vi "Wait For Motion.vi"(8 "error in":errorcluster, 10 "Axes":string[](array[string])=["X", "Y", "Z", "U"], 11 "Gantry in":refnum<class "Gantry.lvclass">) -> (0 "error out":errorcluster, 3 "Gantry out":refnum<class "Gantry.lvclass">)   [LabVIEW 2026, in "Gantry.lvclass"]
uses:
  Gantry.lvclass
  <instrlib>/Aerotech Automation1/Aerotech Automation1.lvlib
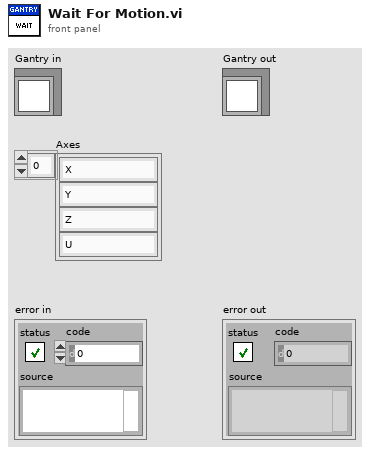
[diagram p1: front panel]
types:
  T1 = typedef "Virtual Modes.ctl" = enum16{"Nonvirtual", "Virtual"}
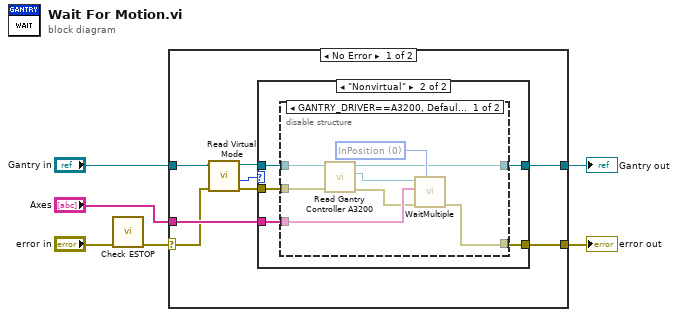
[diagram p0: block diagram]
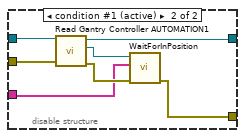
[diagram p3: hidden frame]
diagram:
  n1 = call "Check ESTOP.vi"("error in"="error in") -> ("error out"=w2:errorcluster)  [unwired: 10 in]
  n2 = case shown="No Error" w2 {
    selector: w2 -> [w8 w38]
    tunnel: [w12 w38] -> w6
    tunnel: [w14 w37] -> w5
    tunnel: "Gantry in" -> [w11 w37]
    tunnel: "Axes" -> [w13 _]
    frame No Error {
      n3 = call-dynamic "Read Virtual Mode.vi"("error in (no error)"=w8, "Gantry in"=w11) -> ("error out"=w7:errorcluster, "Virtual Mode"=w9:T1, "Gantry out"=w10:refnum<class "Gantry.lvclass">)  [unwired: 6 in, 1 out]
      n4 = case shown="\"Nonvirtual\"" w9 {
        tunnel: w10 -> [w16 w19]
        tunnel: [w16 w17] -> w14
        tunnel: w13 -> [_ w21]
        tunnel: w7 -> [w15 w18]
        tunnel: [w15 w20] -> w12
        frame "Virtual" {
        }
        frame "Nonvirtual" {
          n5 = disable-structure shown="GANTRY_DRIVER==A3200, Default" {
            disable-tunnel: w21 -> [w29 w31]
            disable-tunnel: [w28 w30] -> w20
            disable-tunnel: w19 -> [w26 w34]
            disable-tunnel: w18 -> [w25 w32]
            disable-tunnel: [w24 w33] -> w17
            frame condition #0 {
              w27 = 0 items=["InPosition", "MoveDone"] ("wait option?")
              n6 = call "Read Gantry Controller A3200.vi"("error in (no error)"=w25, "Gantry in"=w26) -> ("error out"=w23:errorcluster, "A3200 controller out"=w22:refnum<k24>, "Gantry out"=w24:refnum<class "Gantry.lvclass">)  [unwired: 7 in]
              n7 = call "WaitMultiple.vi"("wait option?"=w27, "error in (no error)"=w23, "axis names"=w29, "controller in"=w22) -> ("error out"=w28:errorcluster)  [unwired: 5 in, 2 out]
            }
            frame condition #1 (active) {
              n8 = call "Read Gantry Controller AUTOMATION1.vi"("error in (no error)"=w32, "Gantry in"=w34) -> ("error out"=w35:errorcluster, "Controller AUTOMATION1"=w36:refnum<k24>, "Gantry out"=w33:refnum<class "Gantry.lvclass">)  [unwired: 7 in]
              n9 = call <instrlib>:"WaitForInPosition.vi"("error in (no error)"=w35, "axes"=w31, "Controller Refnum"=w36) -> ("error out"=w30:errorcluster)  [unwired: 7 in, 1 out]
            }
          }
        }
      }
    }
    frame Error {
    }
  }
  "error out" <- w6
  "Gantry out" <- w5
